vi "Actor Core.vi"(8 "error in":errorcluster, 11 "Analog-Output in":refnum<class "Analog-Output.lvclass">) -> (0 "error out":errorcluster, 3 "Actor out":refnum<class "Actor.lvclass">)   [LabVIEW 2019, in "Analog-Output.lvlib" / "Analog-Output.lvclass"]
doc: "The instrument actor core is only here to distribute panel resolution settings to children classes."
uses:
  Library/Analog-Output.lvclass
  builds/Engine/Actor Framework.lvlibp/1abvi3w/vi.lib/ActorFramework/Actor/Actor.lvclass
  Custom Controls/Settings.ctl
  Library/Analog-Output.lvclass/Analog-Output.ctl
  Analog-Output Messages/Set Voltage Msg/Set Voltage Msg.lvclass/Set Voltage Msg.ctl
  Analog-Output Messages/Write Active Channel Msg/Write Active Channel Msg.lvclass/Write Active Channel Msg.ctl
  Accessors/Write Channel.vi
  Accessors/Write Measured Table.vi
  Accessors/Write Settings.vi
  builds/Engine/Actor Framework.lvlibp/1abvi3w/vi.lib/ActorFramework/Message Enqueuer/Enqueue.vi
  Analog-Output Messages/Set Voltage Msg/Set Voltage Msg.lvclass
  Analog-Output Messages/Write Active Channel Msg/Write Active Channel Msg.lvclass
  builds/Instruments/Instruments.lvlibp/Library/Instruments.lvclass
  C:/Users/Public/Documents/Development/builds/Instruments/Instruments.lvlibp/Library/Instruments.lvclass
panel:
  in  "Active Device":u16(ring)
  out "Measured Table":i32(listbox)
  in  "Settings":T1
  in  "Channel":u16(ring)
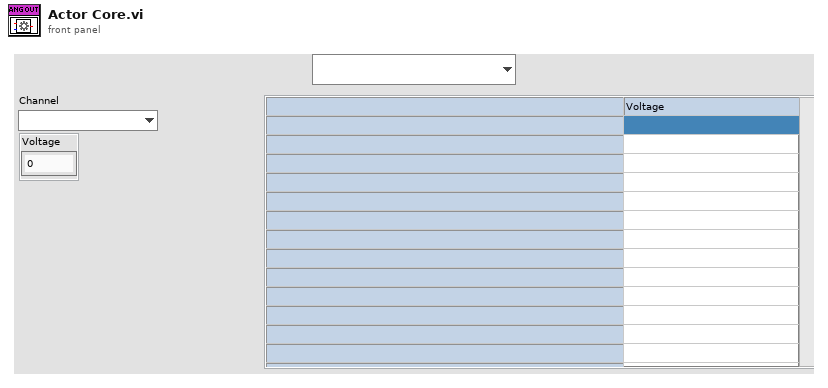
[diagram p1: front panel]
types:
  T1 = typedef "Analog-Output.lvlib/Analog-Output.lvclass/Settings.ctl" = cluster{"Voltage":dbl}
  T2 = cluster{"Pnl Actor":refnum<event-registration>, "Event Registration Refnum":refnum<event-registration>}
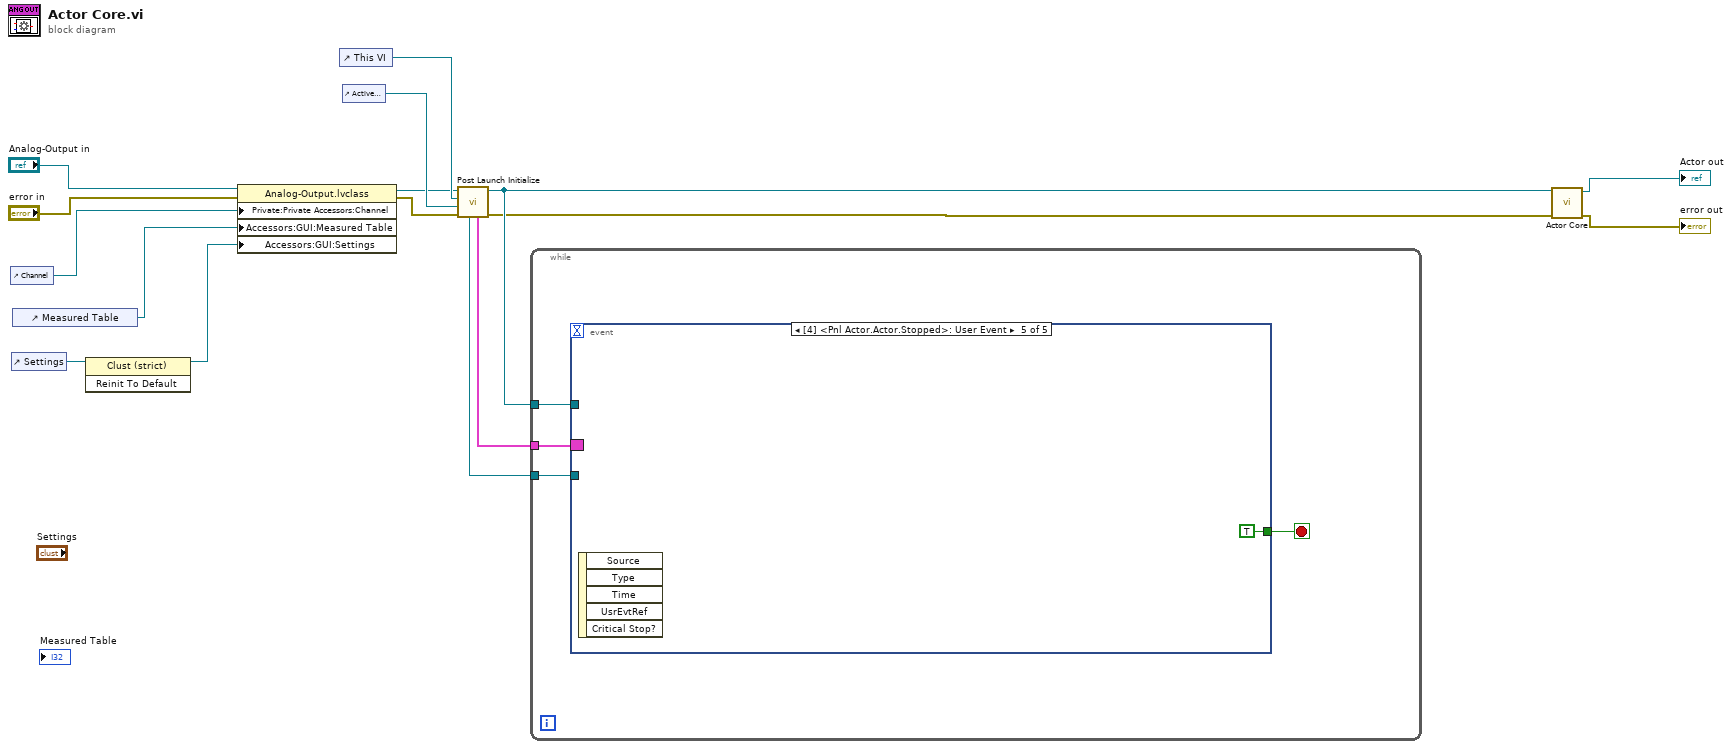
[diagram p0: block diagram]
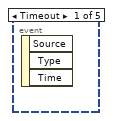
[diagram p2: hidden frame]
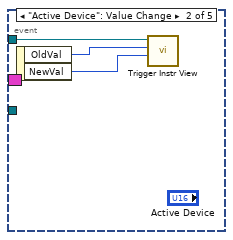
[diagram p3: hidden frame]
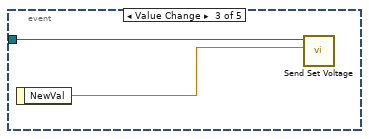
[diagram p4: hidden frame]
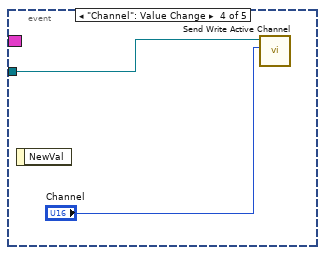
[diagram p5: hidden frame]
diagram:
  n1 = control-ref of="Channel"() -> (w5:refnum<vi>)
  n2 = control-ref of="Settings"() -> (w2:refnum<vi>)
  n3 = control-ref of="Measured Table"() -> (w4:refnum<vi>)
  n4 = invoke class="Clust (strict)" method="Reinit To Default"(reference=w2) -> (reference out=w1:refnum<vi>)  [unwired: 2 in, 2 out]
  n5 = property class="Analog-Output.lvclass"(reference="Analog-Output in", error in="error in", "Private:Private Accessors:Channel"=w5, "Accessors:GUI:Measured Table"=w4, "Accessors:GUI:Settings"=w1) -> (reference out=w9:refnum<class "Analog-Output.lvclass">, error out=w7:errorcluster)
  n6 = control-ref of="This VI"() -> (w10:refnum<vi>)
  n7 = control-ref of="Active Device"() -> (w11:refnum<vi>)
  n8 = call "Post Launch Initialize.vi"("error in"=w7, "Active Device"=w11, "GUI Reference"=w10, "Instruments in"=w9) -> ("error out"=w3:errorcluster, "Instruments out"=w12:refnum<class "Analog-Output.lvclass">, "Registered Events"=w14:T2, "Self Enqueuer"=w13:refnum<class "Message Enqueuer.lvclass">)  [unwired: 4 in]
  n9 = while {
    tunnel: w14 -> [w20]
    tunnel: w13 -> [w19]
    tunnel: w12 -> [w18]
    stop <- w17 stop-if-true
    n10 = event shown="[4] <Pnl Actor.Actor.Stopped>: User Event" {
      selector: w20 -> [_ _ _ _ _]
      dyn-events: _ -> [_ _ _ _ _]
      timeout: _ -> [_ _ _ _ _]
      tunnel: w19 -> [_ _ w25 w26 _]
      tunnel: w18 -> [_ w21 _ _ _]
      tunnel: [_ _ _ _ TRUE ("Discard?")] -> w17
      event Timeout {
        n11 = event-data() -> ()  [unwired: 1 in, 3 out]
      }
      event "Active Device": Value Change {
        n12 = event-data() -> ("OldVal"=w23:u16, "NewVal"=w22:u16)  [unwired: 1 in]
        n13 = call "Trigger Instr View.vi"("New Value"=w22, "Old Value"=w23, "Instruments in"=w21) -> ()  [unwired: 7 in, 2 out]
      }
      event Value Change {
        n14 = event-data() -> ("NewVal"=w24:dbl)  [unwired: 1 in]
        n15 = call "Send Set Voltage.vi"("Voltage"=w24, "Message Enqueuer"=w25) -> ()  [unwired: 8 in, 2 out]
      }
      event "Channel": Value Change {
        n16 = event-data() -> ()  [unwired: 1 in, 1 out]
        n17 = call "Send Write Active Channel.vi"("Active Channel"="Channel", "Message Enqueuer"=w26) -> ()  [unwired: 8 in, 2 out]
      }
      event User Event {
        n18 = event-data() -> ()  [unwired: 1 in, 5 out]
      }
    }
  }
  n19 = call-parent "Actor Core.vi"("error in"=w3, "Instruments in"=w12) -> ("error out"=→"error out":errorcluster, "Actor out"=→"Actor out":refnum<class "Actor.lvclass">)  [unwired: 8 in]
